vi "ProcessMouseEvents.vi"(6 "Reset on True":bool, 8 "error in (no error)":errorcluster, 9 "Dots per inch":i32, 10 "byte order (0:big-endian, network order)":T1(ring)=enum."little-endian", 11 "Byte Stream File in":refnum<file>) -> (0 "error out":errorcluster, 1 "X Position (um)":dbl, 2 "Y Position (um)":dbl, 3 "Byte Stream File out":refnum<file>, 4 "Left Click Down":bool, 5 "Right Click Down":bool)   [LabVIEW 2015]
uses:
  input_event.ctl
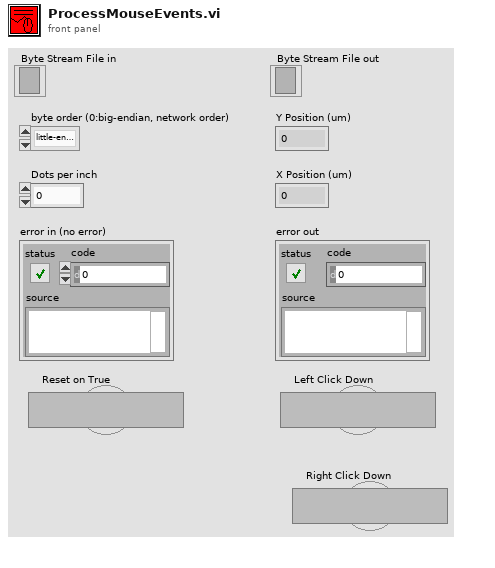
[diagram p1: front panel]
types:
  T1 = enum16{"big-endian, network order", "native, host order", "little-endian"}
  T2 = typedef "input_event.ctl" = cluster{"timeval":cluster{i32, i32}, "type":u16, "code":u16, "value":u32}
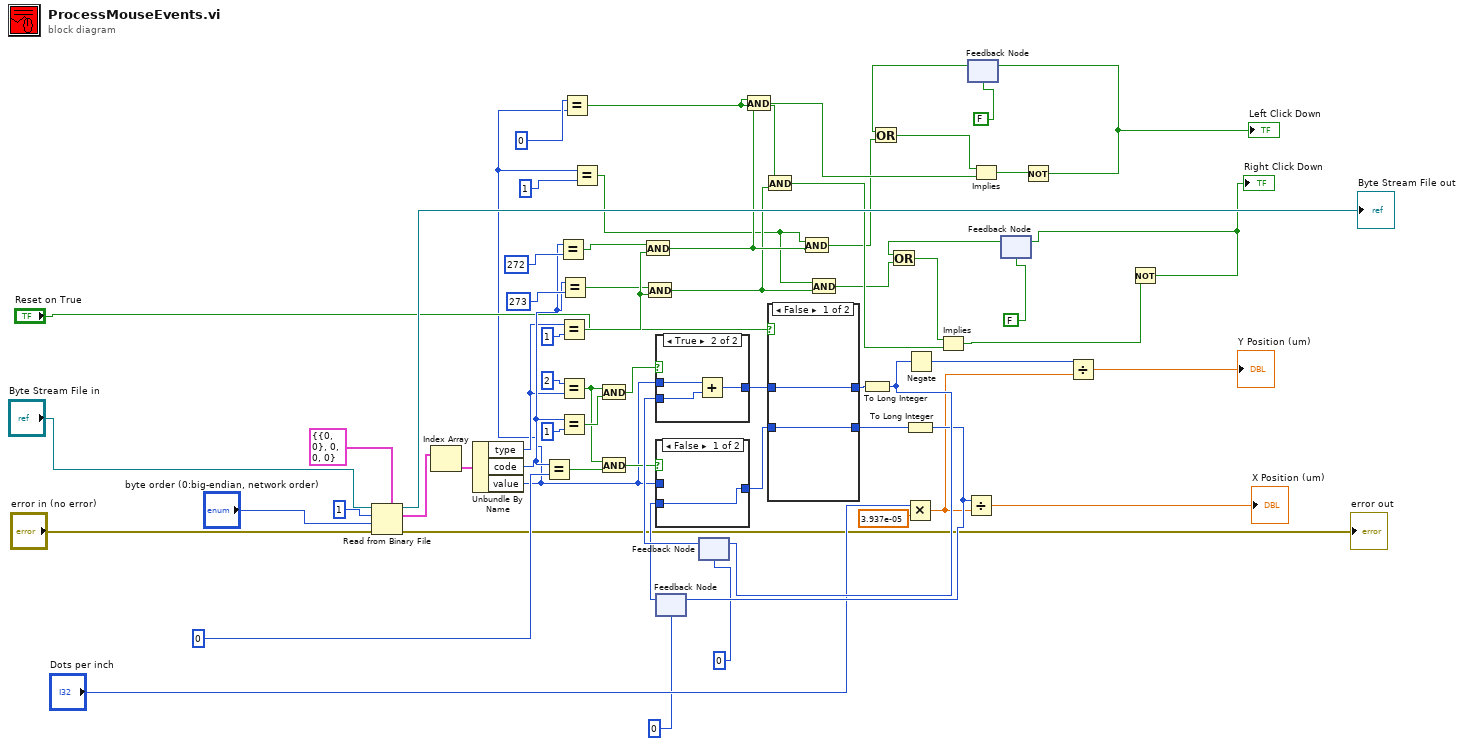
[diagram p0: block diagram]
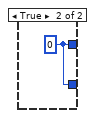
[diagram p3: hidden frame]
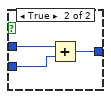
[diagram p4: hidden frame]
diagram:
  n1 = Read from Binary File(5:T2 {"timeval"={0, 0}, "type"=0, "code"=0, "value"=0} ("input_event"), 8:"error in (no error)", 9:"byte order (0:big-endian, network order)", 10:1 ("count (1)"), 11:"Byte Stream File in") -> (0:→"error out":errorcluster, 2:w35:T2[], 3:→"Byte Stream File out":refnum<file>)  [unwired: 1 in, 1 out]
  n2 = Index Array(array=w35) -> (element=w36:T2)  [unwired: 1 in]
  n3 = Unbundle By Name(w36) -> ("type"=w24:u16, "code"=w27:u16, "value"=w5:u32)
  n4 = Equal?(x=w27, y=0) -> (x = y?=w44:bool)
  n5 = Equal?(x=w27, y=272) -> (x = y?=w23:bool)
  n6 = Equal?(x=w24, y=1) -> (x = y?=w26:bool)
  n7 = Equal?(x=2, y=w24) -> (x = y?=w49:bool)
  n8 = Equal?(x=w27, y=1) -> (x = y?=w50:bool)
  n9 = Equal?(x=w27, y=273) -> (x = y?=w9:bool)
  n10 = Equal?(x=0, y=w5) -> (x = y?=w8:bool)
  n11 = Equal?(x=w5, y=1) -> (x = y?=w2:bool)
  n12 = And(x=w49, y=w50) -> (x .and. y?=w51:bool)
  n13 = And(x=w49, y=w44) -> (x .and. y?=w45:bool)
  n14 = And(x=w23, y=w26) -> (x .and. y?=w7:bool)
  n15 = And(x=w9, y=w26) -> (x .and. y?=w3:bool)
  n16 = feedback #1(0) -> (w48:i32)
  n17 = case shown="False" w45 {
    tunnel: w5 -> [_ w67]
    tunnel: w48 -> [w64 w66]
    tunnel: [w64 w65] -> w47
    frame False {
    }
    frame True {
      n18 = Add(x=w67, y=w66) -> (x+y=w65:u32)
    }
  }
  n19 = feedback #2(0) -> (w53:i32)
  n20 = case shown="True" w51 {
    tunnel: w5 -> [_ w71]
    tunnel: [w68 w69] -> w52
    tunnel: w53 -> [w68 w70]
    frame False {
    }
    frame True {
      n21 = Add(x=w71, y=w70) -> (x+y=w69:u32)
    }
  }
  n22 = And(x=w8, y=w7) -> (x .and. y?=w12:bool)
  n23 = And(x=w8, y=w3) -> (x .and. y?=w10:bool)
  n24 = case shown="False" "Reset on True" {
    tunnel: w47 -> [w73 _]
    tunnel: [w73 w74] -> w60
    tunnel: w52 -> [w72 _]
    tunnel: [w72 w74] -> w59
    frame False {
    }
    frame True {
      w74 = 0
    }
  }
  n25 = And(x=w2, y=w7) -> (x .and. y?=w4:bool)
  n26 = And(x=w2, y=w3) -> (x .and. y?=w1:bool)
  n27 = To Long Integer(number=w59) -> (32bit integer=w62:i32)
  n28 = feedback-in #2(w62) -> ()
  n29 = To Long Integer(number=w60) -> (32bit integer=w61:i32)
  n30 = feedback-in #1(w61) -> ()
  n31 = Multiply(x="Dots per inch", y=3.937e-05) -> (x*y=w56:dbl)
  n32 = Negate(x=w62) -> (-x=w63:i32)
  n33 = Divide(x=w61, y=w56) -> (x/y=→"X Position (um)":dbl)
  n34 = feedback #3(FALSE) -> (w20:bool)
  n35 = Or(x=w20, y=w4) -> (x .or. y?=w19:bool)
  n36 = Implies(1:w12, 2:w19) -> (0:w18:bool)
  n37 = feedback #4(FALSE) -> (w17:bool)
  n38 = Or(x=w17, y=w1) -> (x .or. y?=w16:bool)
  n39 = Implies(1:w10, 2:w16) -> (0:w14:bool)
  n40 = Not(x=w18) -> (.not. x?=w15:bool)
  "Left Click Down" <- w15
  n41 = feedback-in #3(w15) -> ()
  n42 = Divide(x=w63, y=w56) -> (x/y=→"Y Position (um)":dbl)
  n43 = Not(x=w14) -> (.not. x?=w13:bool)
  "Right Click Down" <- w13
  n44 = feedback-in #4(w13) -> ()
